vi "Pcre2JitStackFree8.vi"(8 "error in":errorcluster, 11 "pJitStack":u64 format="%.0x") -> (0 "error out":errorcluster)   [LabVIEW 2021, in "libpcre2-8.lvlib"]
uses:
  libpcre2-8.lvlib
  libpcre2-8-x32.dll
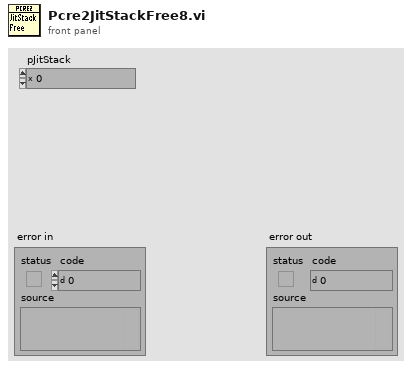
[diagram p1: front panel]
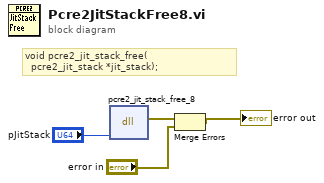
[diagram p0: block diagram]
diagram:
  # "void pcre2_jit_stack_free(\n  pcre2_jit_stack *jit_stack);"
  n1 = dll-call lib="libpcre2-8-x*.dll" fn="pcre2_jit_stack_free_8"("jit_stack"="pJitStack") -> (error out=w3:errorcluster)  [unwired: 5 in, 1 out]
  n2 = Merge Errors(w3, "error in") -> (→"error out":errorcluster)
